vi "gerador de trajetoria.vi"(0 "passar pelos\npontos:":cluster{"X":dbl, "Y":dbl}[](array[cluster]), 1 "x inicial":dbl, 2 "x final":dbl, 3 "Número de passos":u32) -> (7 "pontos\ninterpolados":cluster{"X":dbl, "Y":dbl}[](array[cluster]))   [LabVIEW 2016]
uses:
  <vilib>/gmath/NI_Gmath.lvlib
panel:
  out "XY Graph":cluster{"X":dbl, "Y":dbl}[](graph)
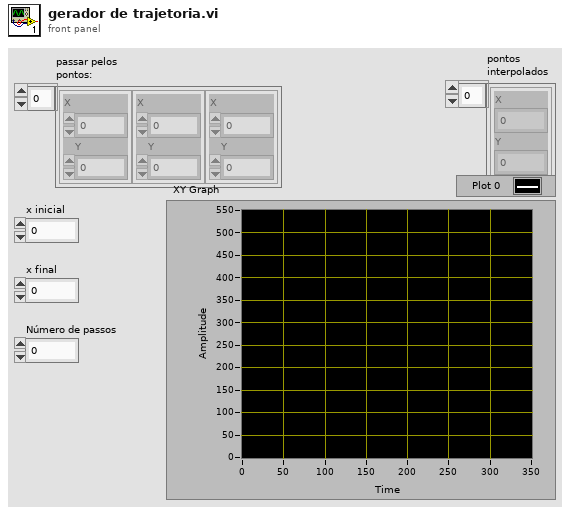
[diagram p1: front panel]
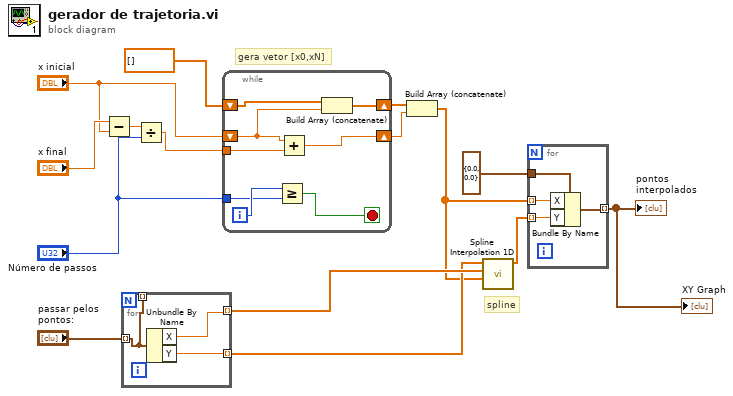
[diagram p0: block diagram]
diagram:
  # "spline"
  # "gera vetor [x0,xN]"
  n1 = Subtract(x="x final", y="x inicial") -> (x-y=w14:dbl)
  n2 = for {
    tunnel: "passar pelos\npontos:" -> [w16] mode=indexing
    tunnel: [w18] -> w6 mode=indexing
    tunnel: [w17] -> w5 mode=indexing
    tunnel: [w16] -> _ mode=indexing
    n3 = Unbundle By Name(w16) -> ("X"=w18:dbl, "Y"=w17:dbl)
  }
  n4 = Divide(x=w14, y="Número de passos") -> (x/y=w13:dbl)
  n5 = while {
    shift-right: [w19] -> w8
    shift-left: "x inicial" -> [w20]
    tunnel: w13 -> [w26]
    tunnel: "Número de passos" -> [w23]
    shift-right: [w22] -> w9
    shift-left: dbl[] [] -> [w21]
    i -> [w24]
    stop <- w25 stop-if-true
    n6 = Greater Or Equal?(x=w24, y=w23) -> (x >= y?=w25:bool)
    n7 = Add(x=w20, y=w26) -> (x+y=w19:dbl)
    n8 = Build Array (concatenate)(w21, w20) -> (w22:dbl[])
  }
  n9 = Build Array (concatenate)(w9, w8) -> (w3:dbl[])
  n10 = call <vilib>:"Spline Interpolation 1D.vi"("xi"=w3, "X"=w6, "Y"=w5) -> ("yi"=w2:dbl[])  [unwired: 6 in, 2 out]
  n11 = for {
    tunnel: cluster{"X":dbl, "Y":dbl} {"X"=0.0, "Y"=0.0} ("ponto") -> [w30]
    tunnel: w3 -> [w29] mode=indexing
    tunnel: w2 -> [w28] mode=indexing
    tunnel: [w27] -> w1 mode=indexing
    n12 = Bundle By Name(cluster=w30, "X"=w29, "Y"=w28) -> (w27:cluster{"X":dbl, "Y":dbl})
  }
  "pontos\ninterpolados" <- w1
  "XY Graph" <- w1
